vi "POSITION ARM ANGLE.vi"(0 "motor devref LEFT":T1={"DeviceStatus"={"status"=FALSE, "code"=0, "source"=""}, "Type"=enum."PWM", "PWM"={"PWM Channel"=enum."Invalid", "DeadBand"={"Name"="", "maxPositivePwm"=0, "minPositivePwm"=0, "centerPwm"=0, "maxNegativePwm"=0, "minNegativePwm"=0, "angularRange"=0}}, "CAN"={"Device Number"=0, "SetOutput VI Ref"=variant, "GetOutput VI Ref"=variant, "Enable VI Ref"=variant, "Disable VI Ref"=variant, "Data"=variant}, "Invert"=FALSE, "DIO PWM"={"PWM \"Enable\" Channel"=enum."Invalid", "DIOChannel"=enum."Invalid", "PWM Rate"=0.0}}, 2 "Setpoint LEFT":dbl=515.0, 5 "error in (no error)":errorcluster, 7 "Left PID Constants":T6={"P Gain"=2.0599999999999987, "I Gain"=0.0, "D Gain"=0.20000000000000004, "F Gain"=0.0, "I Zone"=0.0, "Min Output"=-0.1999999999999993, "Max Output"=0.95} {"Max Output" min=-1.0 max=1.0 step=0.01; "Min Output" min=-1.0 max=1.0 step=0.01; "I Zone" step=0.01; "F Gain" step=0.01; "D Gain" step=0.01; "I Gain" step=0.01; "P Gain" min=0.0 step=0.01}) -> (14 "Position LEFT":dbl, 16 "Output LEFT":dbl, 19 "error out":errorcluster)   [LabVIEW 2020]
uses:
  <vilib>/Rock Robotics/WPI/MotorControl/WPI_MotorControlDeviceRef.ctl
  <vilib>/Rock Robotics/WPI/MotorControl/WPI_MotorControlType.ctl
  <vilib>/Rock Robotics/SystemInterfaces/DIO/FPGA_DIOPWMChannel.ctl
  <vilib>/Rock Robotics/WPI/PWM/WPI_PWMDeadband.ctl
  <vilib>/Rock Robotics/SystemInterfaces/DIO/FPGA_DIOChannel.ctl
  <vilib>/Rock Robotics/WPI/ThirdParty/REV Robotics/REVLib/Typedef/Spark MAX Control Type.ctl
panel:
  out "Left PID Chart":T7(graph)={"Sensor Velocity"=515.0147705078125, "Setpoint"=515.0, "Applied Output"=0.01858577227088229}
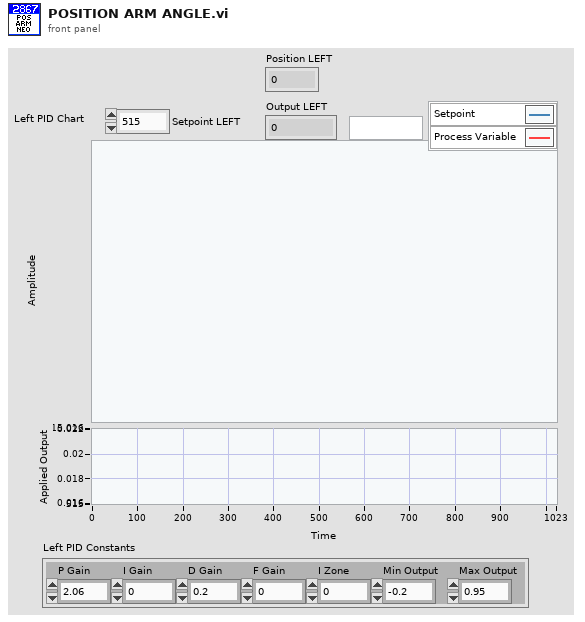
[diagram p1: front panel]
types:
  T1 = typedef "WPI_MotorControlDeviceRef.ctl" = cluster{"DeviceStatus":errorcluster, "Type":T2, "PWM":cluster{"PWM Channel":T3, "DeadBand":T4}, "CAN":cluster{"Device Number":u8, "SetOutput VI Ref":variant, "GetOutput VI Ref":variant, "Enable VI Ref":variant, "Disable VI Ref":variant, "Data":variant}, "Invert":bool, "DIO PWM":cluster{"PWM \"Enable\" Channel":T3, "DIOChannel":T5, "PWM Rate":dbl}}
  T2 = typedef "WPI_MotorControlType.ctl" = enum16{"PWM", "CAN", "DIO PWM"}
  T3 = typedef "FPGA_DIOPWMChannel.ctl" = enum8{"PWM 0", "PWM 1", "PWM 2", "PWM 3", "PWM 4", "PWM 5", "PWM 6", "PWM 7", "PWM 8", "PWM 9", "PWM MXP 0", "PWM MXP 1", "PWM MXP 2", "PWM MXP 3", "PWM MXP 4", "PWM MXP 5", "PWM MXP 6", "PWM MXP 7", "PWM MXP 8", "PWM MXP 9", "Invalid"}
  T4 = typedef "WPI_PWMDeadband.ctl" = cluster{"Name":string, "maxPositivePwm":i32, "minPositivePwm":i32, "centerPwm":i32, "maxNegativePwm":i32, "minNegativePwm":i32, "angularRange":u16}
  T5 = typedef "FPGA_DIOChannel.ctl" = enum8{"DIO 0", "DIO 1", "DIO 2", "DIO 3", "DIO 4", "DIO 5", "DIO 6", "DIO 7", "DIO 8", "DIO 9", "DIO MXP 0", "DIO MXP 1", "DIO MXP 2", "DIO MXP 3", "DIO MXP 4", "DIO MXP 5", "DIO MXP 6", "DIO MXP 7", "DIO MXP 8", "DIO MXP 9", "DIO MXP 10", "DIO MXP 11", "DIO MXP 12", "DIO MXP 13", "DIO MXP 14", "DIO MXP 15", "SPI Port CS1", "SPI Port CS2", "SPI Port CS3", "SPI Port MISO", "SPI Port MOSI", "Invalid"}
  T6 = cluster{"P Gain":dbl, "I Gain":dbl, "D Gain":dbl, "F Gain":dbl, "I Zone":dbl, "Min Output":dbl, "Max Output":dbl}
  T7 = cluster{"Sensor Velocity":dbl, "Setpoint":dbl, "Applied Output":dbl}
  T8 = typedef "Spark MAX Control Type.ctl" = enum16{"Percent VBus", "Voltage", "Velocity", "Position", "Smart Motion", "Current", "Smart Velocity"}
  T9 = cluster{"P Gain":bool, "I Gain":bool, "D Gain":bool, "F Gain":bool, "I Zone":bool, "Min Output":bool, "Max Output":bool}
  T10 = typedef "Spark MAX Status 2 Frame.ctl" = cluster{"Sensor Position":dbl, "IAccum":dbl, "Timestamp":u32}
  T11 = typedef "Spark MAX Status 0 Frame.ctl" = cluster{"Applied Output":dbl, "Faults":T12, "Sticky Faults":T12, "Rsvd":u8, "Status 0 Flags":T13, "Timestamp":u32}
  T12 = typedef "Spark MAX Faults.ctl" = cluster{"Hard Limit Rev":bool, "Hard Limit Fwd":bool, "Soft Limit Fwd":bool, "Soft Limit Rev":bool, "Other Fault":bool, "DRV Fault":bool, "Has Reset?":bool, "CAN RX":bool, "CAN TX":bool, "EEPROM CRC":bool, "Stall":bool, "Sensor Fault":bool, "Motor Type Fault":bool, "IWDT Reset":bool, "Over Current":bool, "Brownout":bool}
  T13 = typedef "Spark MAX Status 0 Flags.ctl" = cluster{"Invert/Brake":bool, "Is Follower":bool}
  T14 = cluster{"Sensor Position":dbl, "Setpoint LEFT":dbl, "Applied Output":dbl}
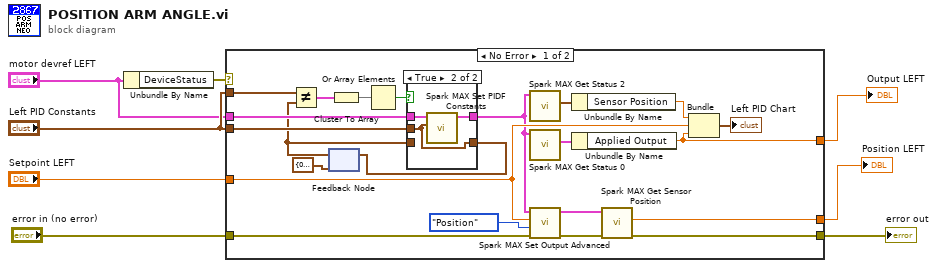
[diagram p0: block diagram]
diagram:
  n1 = Unbundle By Name("motor devref LEFT") -> ("DeviceStatus"=w2:errorcluster)
  n2 = case shown="No Error" w2 {
    tunnel: "motor devref LEFT" -> [w30 _]
    tunnel: "Setpoint LEFT" -> [w29 _]
    tunnel: "Left PID Constants" -> [w28 _]
    tunnel: "Left PID Constants" -> [w27 _]
    tunnel: [w9 _] -> w6
    tunnel: [w14 _] -> w5
    tunnel: "error in (no error)" -> [w13 _]
    tunnel: [w12 _] -> w1
    frame No Error {
      n3 = feedback #1(T6 {"P Gain"=0.0, "I Gain"=0.0, "D Gain"=0.0, "F Gain"=0.0, "I Zone"=0.0, "Min Output"=0.0, "Max Output"=0.0} ("PID Constants")) -> (w22:T6)
      n4 = Not Equal?(x=w27, y=w22) -> (x != y?=w17:T9)
      n5 = Cluster To Array(cluster=w17) -> (array=w18:bool[])
      n6 = Or Array Elements(Boolean array=w18) -> (logical OR=w20:bool)
      n7 = case shown="True" w20 {
        tunnel: w30 -> [w31 w35]
        tunnel: w28 -> [_ w33]
        tunnel: [w32 w33] -> w21
        tunnel: w22 -> [w32 _]
        tunnel: [w31 w34] -> w16
        frame False {
        }
        frame True {
          n8 = call <vilib>:"Spark MAX Set PIDF Constants.vi"("PID Constants"=w33, "MotorControlDeviceRef"=w35) -> ("MotorControlDeviceRef"=w34:T1)  [unwired: 8 in, 1 out]
        }
      }
      n9 = feedback-in #1(w21) -> ()
      n10 = call <vilib>:"Spark MAX Get Status 2.vi"("MotorControlDevRef"=w16) -> ("Stat 2"=w15:T10)  [unwired: 7 in, 3 out]
      n11 = call <vilib>:"Spark MAX Get Status 0.vi"("MotorControlDevRef"=w16) -> ("Status 0"=w26:T11)  [unwired: 7 in, 3 out]
      n12 = call <vilib>:"Spark MAX Set Output Advanced.vi"("error in (no error)"=w13, "Control Mode"=Spark_MAX_Control_Type."Position", "Setpoint"=w29, "MotorControlDevRef"=w16) -> ("error out"=w10:errorcluster, "MotorControlDevRef"=w11:T1)  [unwired: 6 in]
      n13 = Unbundle By Name(w15) -> ("Sensor Position"=w23:dbl)
      n14 = Unbundle By Name(w26) -> ("Applied Output"=w14:dbl)
      n15 = call <vilib>:"Spark MAX Get Sensor Position.vi"("error in (no error)"=w10, "MotorControlDevRef in"=w11) -> ("error out"=w9:errorcluster, "Sensor Position"=w12:dbl)  [unwired: 6 in, 2 out]
      n16 = Bundle("Sensor Position"=w23, "Setpoint LEFT"=w29, "Applied Output"=w14) -> (→"Left PID Chart":T14)  [unwired: 1 in]
    }
    frame Error {
    }
  }
  "Output LEFT" <- w5
  "error out" <- w6
  "Position LEFT" <- w1
